vi "datasutrasmission.vi"(0 "object in":refnum<class "interface.lvclass">, 5 "error in (no error)":errorcluster) -> (14 "object out":refnum<class "interface.lvclass">, 19 "error out":errorcluster)   [LabVIEW 2016, in "interface.lvclass"]
uses:
  interface.lvclass
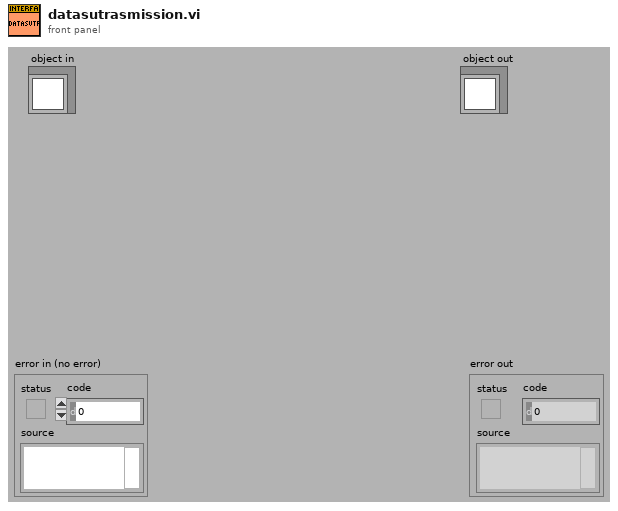
[diagram p1: front panel]
types:
  T1 = cluster{"[0]":string, "[1]":string, "[2]":string, "[3]":string, "[4]":string, "[5]":string, "[6]":string, "[7]":string}
  T2 = cluster{"[0]":string, "[1]":string, "[2]":string, "[3]":string, "[4]":string, "[5]":string, "[6]":string}
  T3 = cluster{"[0]":string, "[1]":string, "[2]":string, "[3]":string, "[4]":string, "[5]":string, "[6]":string, "[7]":string, "[8]":string, "[9]":string, "[10]":string, "[11]":string, "[12]":string, "[13]":string, "[14]":string, "[15]":string, "[16]":string, "[17]":string}
  T4 = cluster{"[0]":string, "[1]":string, "[2]":string, "[3]":string, "[4]":string, "[5]":string, "[6]":string, "[7]":string, "[8]":string, "[9]":string}
  T5 = cluster{"[0]":string, "[1]":string, "[2]":string, "[3]":string, "[4]":string, "[5]":string, "[6]":string, "[7]":string, "[8]":string, "[9]":string, "[10]":string, "[11]":string, "[12]":string, "[13]":string, "[14]":string, "[15]":string, "[16]":string, "[17]":string, "[18]":string, "[19]":string, "[20]":string, "[21]":string, "[22]":string, "[23]":string, "[24]":string, "[25]":string, "[26]":string, "[27]":string, "[28]":string, "[29]":string, "[30]":string, "[31]":string, "[32]":string, "[33]":string, "[34]":string, "[35]":string, "[36]":string}
  T6 = cluster{"[0]":string, "[1]":string, "[2]":string, "[3]":string, "[4]":string, "[5]":string, "[6]":string, "[7]":string, "[8]":string, "[9]":string, "[10]":string, "[11]":string, "[12]":string, "[13]":string, "[14]":string}
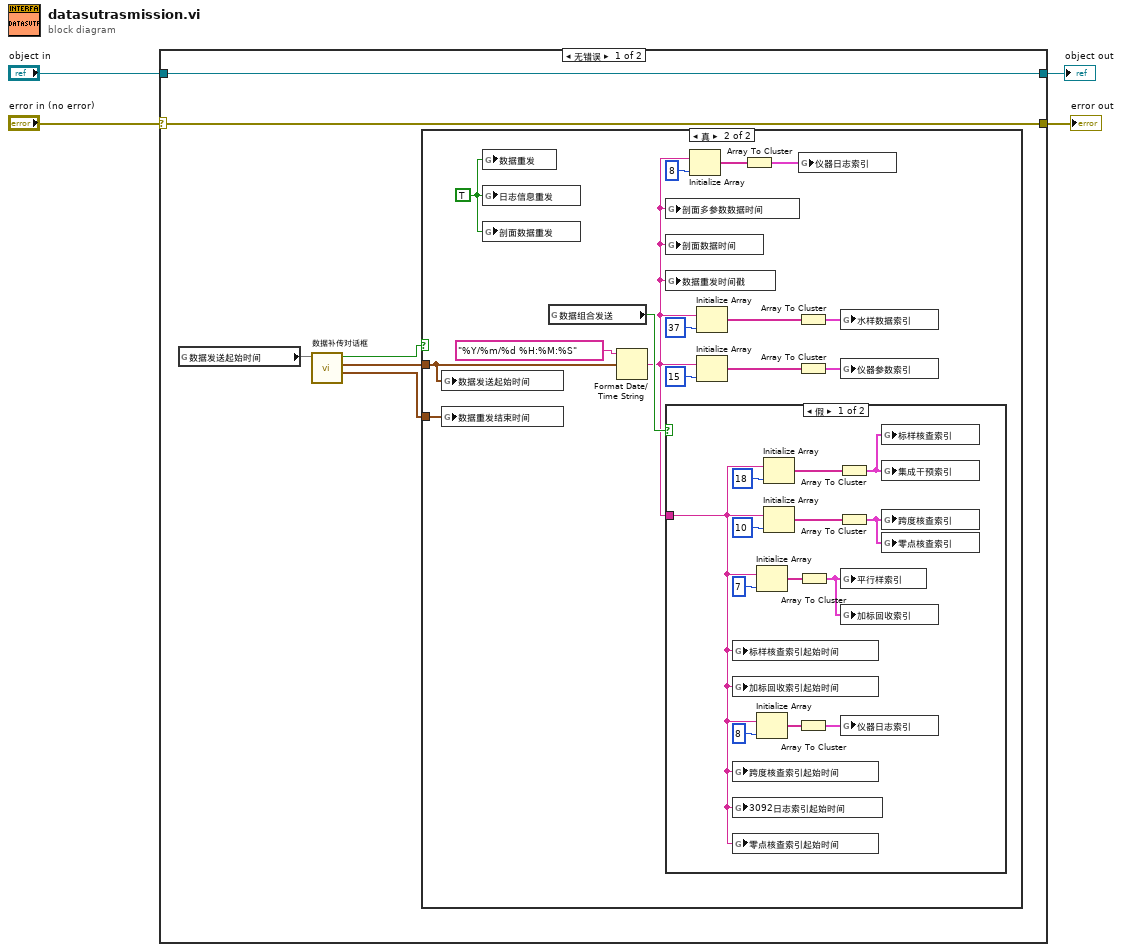
[diagram p0: block diagram]
diagram:
  n1 = case shown="无错误" "error in (no error)" {
    selector: "error in (no error)" -> [w10 w40]
    tunnel: [w10 w40] -> w3
    tunnel: [w9 w39] -> w1
    tunnel: "object in" -> [w9 w39]
    frame No Error {
      n2 = global read "全局1.vi" "数据发送起始时间"() -> (w8)
      n3 = call "数据补传对话框.vi"("起始时间"=w8) -> ("结束时间输出"=w5:timestamp, "起始时间输出"=w6:timestamp, "输出"=w7:bool)  [unwired: 8 in]
      n4 = case shown="真" w7 {
        tunnel: w6 -> [_ w12]
        tunnel: w5 -> [_ w17]
        frame False {
        }
        frame True {
          w11 = TRUE ("数据重发")
          n5 = global write "全局1.vi" "数据发送起始时间"(w12) -> ()
          n6 = global write "断电保存全局.vi" "数据重发结束时间"(w17) -> ()
          n7 = global write "断电保存全局.vi" "数据重发"(w11) -> ()
          n8 = global write "断电保存全局.vi" "日志信息重发"(w11) -> ()
          n9 = global write "断电保存全局.vi" "剖面数据重发"(w11) -> ()
          n10 = global read "断电保存全局.vi" "数据组合发送"() -> (w25:bool)
          n11 = Format Date/Time String(time format string (%c)="%Y/%m/%d %H:%M:%S" ("时间格式字符串(%c)"), seconds (now)=w12) -> (date/time string=w13:string)  [unwired: 1 in]
          n12 = global write "全局 水样时间.vi" "剖面多参数数据时间"(w13) -> ()
          n13 = global write "全局 水样时间.vi" "剖面数据时间"(w13) -> ()
          n14 = global write "断电保存全局.vi" "数据重发时间戳"(w13) -> ()
          n15 = case shown="假" w25 {
            tunnel: w13 -> [w26 _]
            frame False {
              n16 = global write "全局 时间2.vi" "标样核查索引起始时间"(w26) -> ()
              n17 = global write "全局 时间2.vi" "加标回收索引起始时间"(w26) -> ()
              n18 = global write "全局 时间2.vi" "跨度核查索引起始时间"(w26) -> ()
              n19 = global write "全局 时间2.vi" "3092日志索引起始时间"(w26) -> ()
              n20 = global write "全局 时间2.vi" "零点核查索引起始时间"(w26) -> ()
              n21 = Initialize Array(w26, 7 ("维数大小")) -> (w30:string[])
              n22 = Initialize Array(w26, 8 ("维数大小")) -> (w29:string[])
              n23 = Initialize Array(w26, 18 ("维数大小")) -> (w33:string[])
              n24 = Initialize Array(w26, 10 ("维数大小")) -> (w38:string[])
              n25 = Array To Cluster(array=w29) -> (cluster=w28:T1)
              n26 = Array To Cluster(array=w30) -> (cluster=w31:T2)
              n27 = Array To Cluster(array=w33) -> (cluster=w34:T3)
              n28 = Array To Cluster(array=w38) -> (cluster=w37:T4)
              n29 = global write "全局 时间2.vi" "平行样索引"(w31) -> ()
              n30 = global write "全局 时间2.vi" "加标回收索引"(w31) -> ()
              n31 = global write "全局 时间2.vi" "仪器日志索引"(w28) -> ()
              n32 = global write "全局 时间2.vi" "标样核查索引"(w34) -> ()
              n33 = global write "全局 时间2.vi" "集成干预索引"(w34) -> ()
              n34 = global write "全局 时间2.vi" "跨度核查索引"(w37) -> ()
              n35 = global write "全局 时间2.vi" "零点核查索引"(w37) -> ()
            }
            frame True {
            }
          }
          n36 = Initialize Array(w13, 8 ("维数大小")) -> (w16:string[])
          n37 = Initialize Array(w13, 37 ("维数大小")) -> (w22:string[])
          n38 = Initialize Array(w13, 15 ("维数大小")) -> (w18:string[])
          n39 = Array To Cluster(array=w16) -> (cluster=w15:T1)
          n40 = Array To Cluster(array=w22) -> (cluster=w21:T5)
          n41 = Array To Cluster(array=w18) -> (cluster=w19:T6)
          n42 = global write "全局 时间2.vi" "仪器日志索引"(w15) -> ()
          n43 = global write "全局 水样时间.vi" "水样数据索引"(w21) -> ()
          n44 = global write "全局 时间2.vi" "仪器参数索引"(w19) -> ()
        }
      }
    }
    frame Error {
    }
  }
  "error out" <- w3
  "object out" <- w1
